vi "Andeen-Hagerling-2700a-Controler-and-GUI.vi"() -> ()   [LabVIEW 2017]
uses:
  8063e8a4-06c5-440d-83fe-17ec515486ab.vi
  021a5a35-1ebb-4c15-ac28-9b4c8b392a4d.vi
  software/LabVIEW Data/Probes/ah2700a/Andeen-Hagerling 2700/Andeen-Hagerling 2700.lvlib
  <vilib>/measure/NI_MABase.lvlib
panel:
  out "out of":i32
  out "?":string
  in  "Randomization":i32(slide) min=0 max=2 step=1 scale=0.0..2.0
  in  "Freq. Mode":i32(slide)=2 min=0 max=2 step=1 scale=0.0..2.0
  in  "Custom Frequencys":i32[](array[numeric])
  in  "Pressure(torr)":string="7.6E2"
  out "Meas. num.":i32
  in  "Wait between Measure (ms)":u32
  in  "Humidity %":dbl
  in  "Temp in C":dbl
  in  "Freq Reps":i32=4
  in  "append to file?":bool=TRUE
  out "Message":string
  out "Length":u32=66
  out "Remaining":string
  in  "Previous":string
  out "Last Units":string[](array[string])
  out "Last Values":dbl[](array[numeric])
  out "Error Message":string
  out "Measurement":string[](array[string])=["Freq.", "Cap.", "Loss", "Voltage"]
  out "Cap vs Freq":cluster{"X":dbl, "Y":dbl}[](graph)
  out "Tan d vs Freq":cluster{"X":dbl, "Y":dbl}[](graph)
  in  "Sample Label":string="2700A S_ Nt_ __ PEO_ R_"
  in  "Save Folder":string="C:\\Users\\brent_000\\Documents\\Clarke Lab\\labview files\\My 2700A files\\Data\\"
  in  "COMMUTATE\nPARAMETER":i16(slide)=1 scale=0.0..2.0
  in  "Units":dbl=2.0 format="%.2f"
  in  "rms voltage (V)":dbl=0.1 format="%.2f"
  in  "Average":dbl=4.0 format="%.2f"
  in  "AH2700A\nerror in (no error)":errorcluster
  in  "VISA resource (AH2700A)":refnum<visa-resource-name>="GPIB0::28::INSTR"
  # "Brent Boland\nClarke Lab\n2/11/18"
  # "Latest Measurement"
  # "AH2700A Settings"
  # "AH2700A Raw"
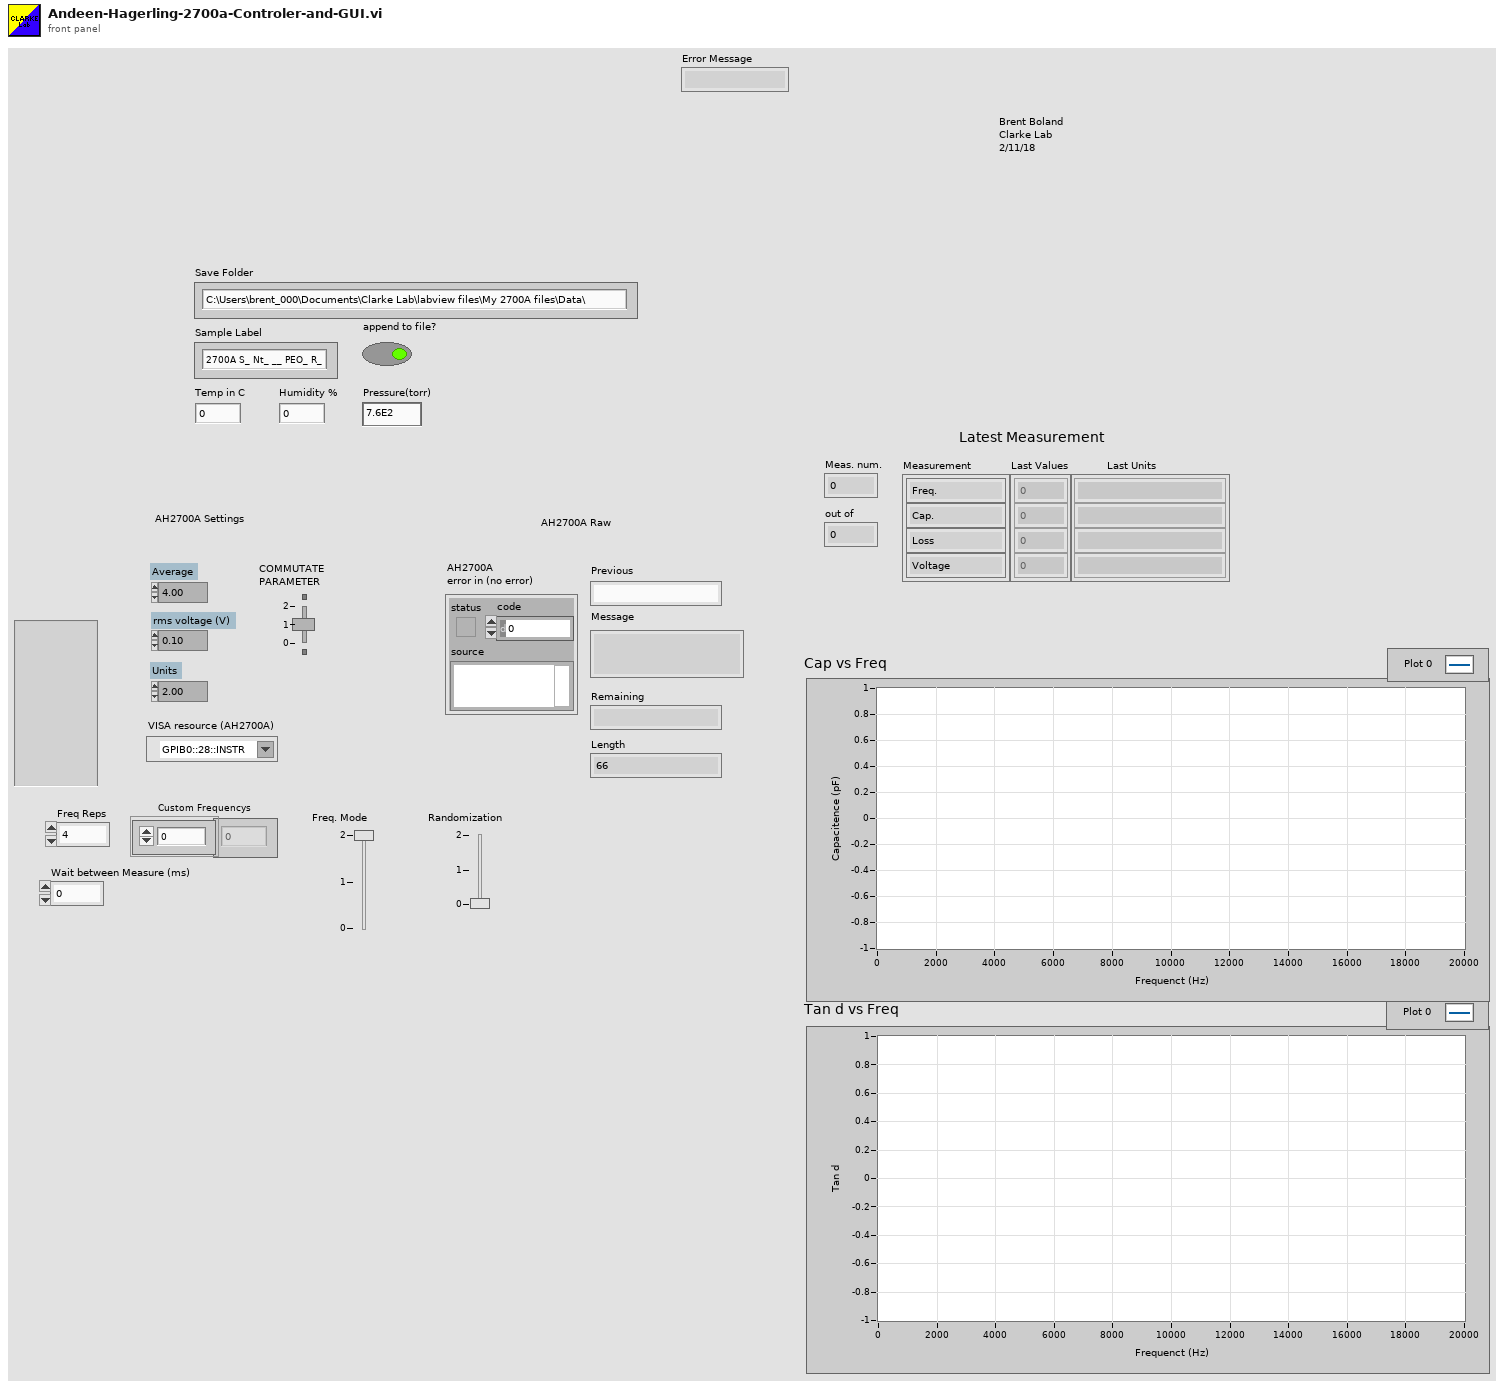
[diagram p1: front panel]
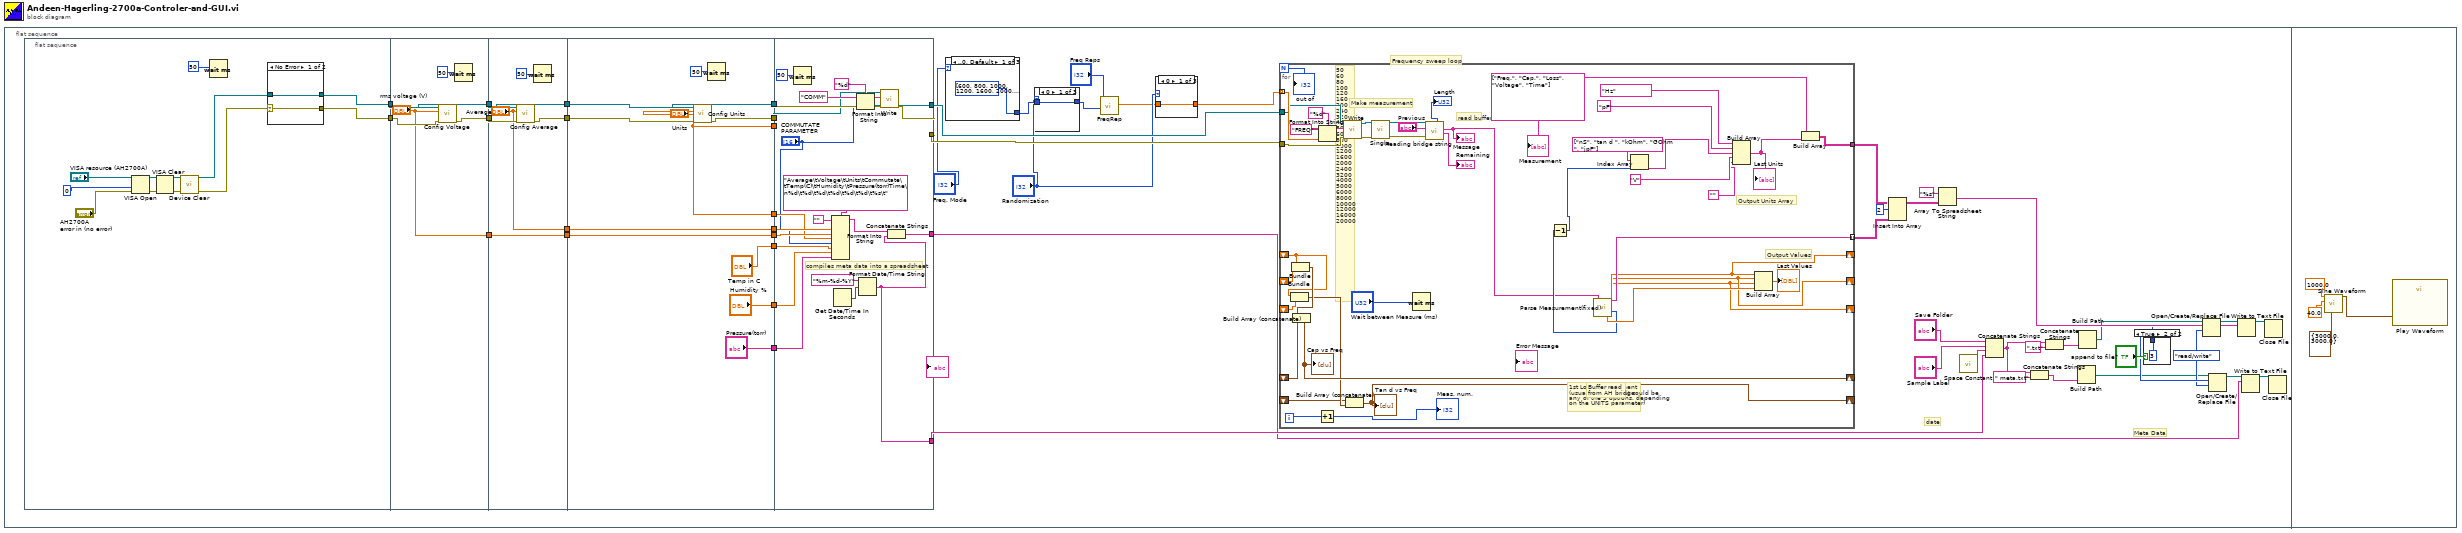
[diagram p0: block diagram]
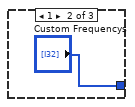
[diagram p2: hidden frame]
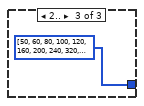
[diagram p3: hidden frame]
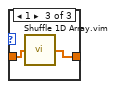
[diagram p5: hidden frame]
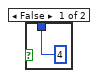
[diagram p6: hidden frame]
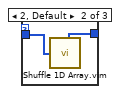
[diagram p7: hidden frame]
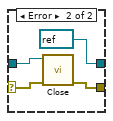
[diagram p9: hidden frame]
diagram:
  # "50\n60\n80\n100\n120\n160\n200\n240\n320\n400\n500\n600\n800\n1000\n1200\n1600\n2000\n2400\n3200\n4000\n5000\n6000\n8000\n10000\n12000\n16000\n20000"
  n1 = flat-sequence {
    frame #0 {
      w15 = enum16{"read/write", "read-only", "write-only"}."read/write" ("access (0:read/write)")
      # "Meta Data"
      # "date"
      # "Frequency sweep loop"
      n2 = flat-sequence {
        tunnel: [w111] -> w52
        tunnel: [w110] -> w51
        tunnel: w52 -> [w133]
        tunnel: [w132] -> w50
        tunnel: [w131] -> w49
        tunnel: w51 -> [w130]
        tunnel: ["rms voltage (V)"] -> w48
        tunnel: w50 -> [w140]
        tunnel: [w139] -> w47
        tunnel: w49 -> [w138]
        tunnel: [w137] -> w46
        tunnel: ["Average"] -> w45
        tunnel: [w134] -> w44
        tunnel: w48 -> [w134]
        tunnel: w47 -> [w151]
        tunnel: w46 -> [w150]
        tunnel: [w149] -> w43
        tunnel: [w148] -> w42
        tunnel: ["Units"] -> w41
        tunnel: [w146] -> w40
        tunnel: w45 -> [w146]
        tunnel: [w145] -> w39
        tunnel: w44 -> [w145]
        tunnel: ["Units"] -> w38
        tunnel: ["Temp in C"] -> w37
        tunnel: ["Humidity %"] -> w36
        tunnel: ["Pressure(torr)"] -> w6
        tunnel: w43 -> [w168]
        tunnel: w42 -> [w170]
        tunnel: [w167] -> w25
        tunnel: [w166] -> w24
        tunnel: w41 -> [_]
        tunnel: w40 -> [w163]
        tunnel: w39 -> [w162]
        tunnel: w38 -> [w161]
        tunnel: [w156] -> w21
        tunnel: [w155] -> w9
        tunnel: w37 -> [w154]
        tunnel: w36 -> [w153]
        tunnel: w6 -> [w152]
        frame #0 {
          n3 = VISA Open(access mode=u32 0, error in (no error)="AH2700A\nerror in (no error)", VISA resource name="VISA resource (AH2700A)") -> (VISA resource name=w117:refnum<visa-resource-name>, error out=w118:errorcluster)  [unwired: 2 in]
          n4 = VISA Clear(VISA resource name=w117, error in (no error)=w118) -> (VISA resource name out=w120:refnum<visa-resource-name>, error out=w121:errorcluster)
          n5 = call "Device Clear.vi"("error in"=w121, "VISA resource name"=w120) -> ("error out"=w113:errorcluster, "VISA resource name out"=w112:refnum<visa-resource-name>)  [unwired: 8 in]
          n6 = Wait (ms)(milliseconds to wait=u32 50 ("millisecond timer value")) -> ()  [unwired: 1 out]
          n7 = case shown="No Error" w113 {
            selector: w113 -> [w122 w125]
            tunnel: w112 -> [w123 w126]
            tunnel: [w123 refnum<visa-resource-name> refnum ("VISA resource name out")] -> w111
            tunnel: [w122 w127] -> w110
            frame No Error {
            }
            frame Error {
              n8 = call "Close.vi"("error in (no error)"=w125, "VISA resource name"=w126) -> ("error out"=w127:errorcluster)  [unwired: 9 in]
            }
          }
        }
        frame #1 {
          n9 = call "Config Voltage.vi"("error in"=w130, "Voltage (15 V)"="rms voltage (V)", "VISA resource name"=w133) -> ("error out"=w131:errorcluster, "VISA resource name out"=w132:refnum<visa-resource-name>)  [unwired: 7 in]
          n10 = Wait (ms)(milliseconds to wait=u32 50 ("millisecond timer value")) -> ()  [unwired: 1 out]
        }
        frame #2 {
          n11 = call "Config Average.vi"("error in"=w138, "Average Exponent (4)"="Average", "VISA resource name"=w140) -> ("error out"=w137:errorcluster, "VISA resource name out"=w139:refnum<visa-resource-name>)  [unwired: 7 in]
          n12 = Wait (ms)(milliseconds to wait=u32 50 ("millisecond timer value")) -> ()  [unwired: 1 out]
        }
        frame #3 {
          n13 = call "Config Units.vi"("error in"=w150, "Units (nS)"="Units", "VISA resource name"=w151) -> ("error out"=w148:errorcluster, "VISA resource name out"=w149:refnum<visa-resource-name>)  [unwired: 7 in]
          n14 = Wait (ms)(milliseconds to wait=u32 50 ("millisecond timer value")) -> ()  [unwired: 1 out]
        }
        frame #4 {
          # "compiles meta data into a spreadsheet"
          n15 = Wait (ms)(milliseconds to wait=u32 50 ("millisecond timer value")) -> ()  [unwired: 1 out]
          n16 = Format Into String(format string="Average\tVoltage\tUnits\tCommutate\tTemp(C)\tHumidity\tPressure(torr)Time\n%d\t%d\t%d\t%d\t%d\t%d\t%s\t", initial string="", w163, w162, w161, "COMMUTATE\nPARAMETER", w154, w153, w152) -> (resulting string=w157:string)  [unwired: 1 in, 1 out]
          n17 = Get Date/Time In Seconds() -> (seconds since 1Jan1904=w159:timestamp)
          n18 = Format Into String(format string="%d", initial string="COMM" ("format string"), "COMMUTATE\nPARAMETER") -> (resulting string=w173:string)  [unwired: 1 in, 1 out]
          n19 = Format Date/Time String(time format string (%c)="%m-%d-%Y", seconds (now)=w159) -> (date/time string=w156:string)  [unwired: 1 in]
          n20 = call "Write.vi"("error in"=w170, "command"=w173, "VISA resource name"=w168) -> ("error out"=w167:errorcluster, "VISA resource name out"=w166:refnum<visa-resource-name>)  [unwired: 7 in]
          n21 = Concatenate Strings(w157, w156) -> (w155:string)
        }
      }
      n22 = case shown="..0, Default" "Freq. Mode" {
        tunnel: [i32[] [600, 800, 1000, 1200, 1600, 2000, 2400, 3200, 4000, 5000, 6000, 8000, 10000, 12000, 16000, 20000] "Custom Frequencys" i32[] [50, 60, 80, 100, 120, 160, 200, 240, 320, 400, 500, 600, 800, 1000, 1200, 1600, 2000, 2400, 3200, 4000, 5000, 6000, 8000, 10000, 12000, 16000, 20000]] -> w7
        frame ..0, Default {
        }
        frame 1 {
        }
        frame 2.. {
        }
      }
      n23 = case shown="0" "Randomization" {
        tunnel: [w62 w64 w65] -> w2
        tunnel: w7 -> [w62 w63 w65]
        frame 0 {
        }
        frame 2, Default {
          n24 = call "Shuffle 1D Array.vim"("array"=w63) -> ("shuffled array"=w64:i32[])  [unwired: 4 in]
        }
        frame 1 {
        }
      }
      n25 = call "FreqRep.vi"("Array"=w2, "Numeric"="Freq Reps") -> ("Array 2"=w4:dbl[])  [unwired: 9 in]
      n26 = case shown="0" "Randomization" {
        tunnel: w4 -> [w56 w57 w59]
        tunnel: [w56 w57 w58] -> w3
        frame 0 {
        }
        frame 2, Default {
        }
        frame 1 {
          n27 = call "Shuffle 1D Array.vim"("array"=w59) -> ("shuffled array"=w58:dbl[])  [unwired: 4 in]
        }
      }
      n28 = for {
        N -> [w66]
        tunnel: w3 -> [w106] mode=indexing
        tunnel: w24 -> [w105]
        tunnel: w25 -> [w104]
        tunnel: [w90] -> w32
        tunnel: [w89] -> w33 mode=indexing
        shift-right: [w82] -> _
        shift-left: _ -> [w74]
        shift-right: [w81] -> _
        shift-left: _ -> [w79]
        shift-right: [w80] -> _
        shift-left: _ -> [w75]
        shift-right: [w77] -> _
        shift-left: _ -> [w76]
        shift-right: [w72] -> _
        shift-left: _ -> [w71]
        i -> [w68]
        w92 = string[] ["Freq.", "Cap.", "Loss", "Voltage", "Time"]
        # "Make measurement"
        # "Output Values"
        # "Output Units Array"
        # "1st Loss Measurement \n(usually, tan d , but could be\nany of the 5 options, depending\non the UNITS parameter)"
        # "Buffer read \nfrom AH bridge"
        # "read buffer"
        n29 = Bundle("Frequency"=w74, "Loss"=w75) -> (w73:cluster{"Frequency":dbl, "Loss":dbl})  [unwired: 1 in]
        n30 = Bundle("Frequency"=w74, "Capacitance"=w79) -> (w78:cluster{"Frequency":dbl, "Capacitance":dbl})  [unwired: 1 in]
        n31 = Build Array (concatenate)(w76, w78) -> (w77:cluster{"Frequency":dbl, "Capacitance":dbl}[])
        "Cap vs Freq" <- w77
        n32 = Increment(x=w68) -> (x+1=→"Meas. num.":i32)
        n33 = Format Into String(format string="%d", initial string="FREQ" ("format string"), w106) -> (resulting string=w109:string)  [unwired: 1 in, 1 out]
        n34 = call "Write.vi"("error in"=w104, "command"=w109, "VISA resource name"=w105) -> ("error out"=w97:errorcluster, "VISA resource name out"=w98:refnum<visa-resource-name>)  [unwired: 7 in]
        n35 = Build Array (concatenate)(w71, w73) -> (w72:cluster{"Frequency":dbl, "Loss":dbl}[])
        "Tan d vs Freq" <- w72
        n36 = call "Single.vi"("error in"=w97, "VISA resource name"=w98) -> ("error out"=w87:errorcluster, "VISA resource name out"=w88:refnum<visa-resource-name>)  [unwired: 8 in]
        n37 = Wait (ms)(milliseconds to wait="Wait between Measure (ms)") -> ()  [unwired: 1 out]
        n38 = call "Reading bridge string.vi"("error in"=w87, "Previous"="Previous", "VISA in"=w88) -> ("Remaining"=→"Remaining":string, "Message"=w84:string, "Length"=→"Length":u32)  [unwired: 4 in, 2 out]
        "Message" <- w84
        n39 = call "Parse Measurement(fixed).vi"("Measurement Line"=w84) -> ("Voltage"=w100:dbl, "Measure String Array"=w89:string[], "Frequency"=w82:dbl, "Capacitance"=w81:dbl, "Loss"=w80:dbl, "Units"=w95:i32)  [unwired: 12 in, 1 out]
        n40 = Decrement(x=w95) -> (x-1=w96:i32)
        n41 = Index Array(array=string[] ["nS", "tan d ", "kOhm", "GOhm ", "jpF"], index=w96) -> (element=w93:string)
        n42 = Build Array("Hz", "pF", w93, "V", "") -> (w91:string[])
        "Last Units" <- w91
        n43 = Build Array(w82, w81, w80, w100) -> (→"Last Values":dbl[])
        n44 = Build Array(w92, w91) -> (w90:string[][])
        "Measurement" <- w92
        "out of" <- w66
      }
      n45 = Insert Into Array(array=w32, index (row)=2, new element=w33) -> (w34:string[][])  [unwired: 1 in]
      n46 = Array To Spreadsheet String(array=w34, 3:"%s" ("format string")) -> (spreadsheet string=w30:string)  [unwired: 1 in]
      n47 = call <vilib>:"Space Constant.vi"() -> ("String"=w20:string)
      n48 = Concatenate Strings("Save Folder", "Sample Label", w20, w21) -> (w18:string)
      n49 = Concatenate Strings(w18, " meta.txt" ("string")) -> (w13:string)
      n50 = Concatenate Strings(w18, ".txt" ("string")) -> (w14:string)
      n51 = Build Path(name or relative path=w13) -> (appended path=w8:path)  [unwired: 1 in]
      n52 = Build Path(name or relative path=w14) -> (appended path=w12:path)  [unwired: 1 in]
      n53 = case shown="True" "append to file?" {
        tunnel: [4 3] -> w16
        frame False {
        }
        frame True {
        }
      }
      n54 = Open/Create/Replace File(file path (use dialog)=w12, operation (0:open)=w16, access (0:read/write)=w15) -> (refnum out=w29:refnum<file>)  [unwired: 3 in, 2 out]
      n55 = Open/Create/Replace File(file path (use dialog)=w8, operation (0:open)=w16, access (0:read/write)=w15) -> (refnum out=w10:refnum<file>)  [unwired: 3 in, 2 out]
      n56 = Write to Text File(file (use dialog)=w29, text=w30) -> (refnum out=w31:refnum<file>)  [unwired: 2 in, 2 out]
      n57 = Write to Text File(file (use dialog)=w10, text=w9) -> (refnum out=w11:refnum<file>)  [unwired: 2 in, 2 out]
      n58 = Close File(refnum=w31) -> ()  [unwired: 1 in, 2 out]
      n59 = Close File(refnum=w11) -> ()  [unwired: 1 in, 2 out]
    }
    frame #1 {
      n60 = call <vilib>:"Sine Waveform.vi"("sampling info"=cluster{"#s":dbl, "Fs":dbl} {"#s"=3000.0, "Fs"=3000.0}, "amplitude"=40.0, "frequency"=1000.0) -> ("signal out"=w177:waveform(dbl))  [unwired: 7 in, 1 out]
      n61 = call "Play Waveform"("Data"=w177) -> ()  [unwired: 18 in, 1 out]
    }
  }
